vi "ReadTestConfig.vi"(11 "Model":string) -> (3 "TestItemsOut":string[][](table))   [LabVIEW 2009]
uses:
  <vilib>/Utility/file.llb/Read From Spreadsheet File (string).vi
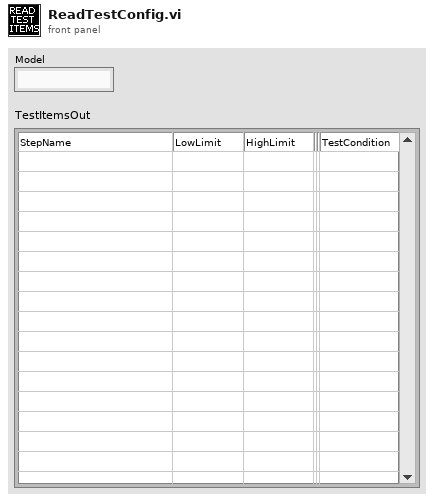
[diagram p1: front panel]
types:
  T1 = enum32{"invalid app kind", "Development System", "Run Time System", "Student Edition", "Embedded LabVIEW", "Evaluation", "Custom"}
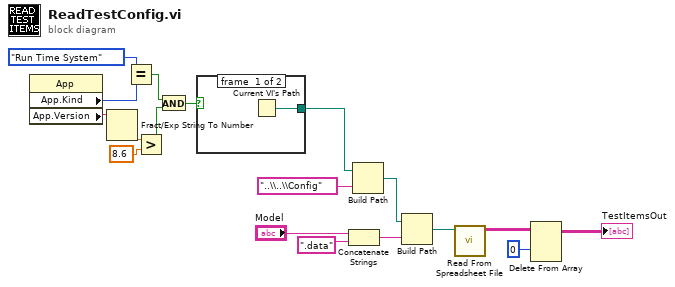
[diagram p0: block diagram]
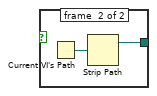
[diagram p2: hidden frame]
diagram:
  n1 = property class="App"() -> ("App.Kind"=w4:T1, "App.Version"=w5:string)  [unwired: 2 in, 2 out]
  n2 = Fract/Exp String To Number(string=w5) -> (number=w6:dbl)  [unwired: 4 out]
  n3 = Equal?(x=T1."Run Time System" ("y"), y=w4) -> (x = y?=w7:bool)
  n4 = Greater?(x=w6, y=8.6) -> (0:w8:bool)
  n5 = And(x=w7, y=w8) -> (x .and. y?=w2:bool)
  n6 = case shown="真" w2 {
    tunnel: [w19 w21] -> w17
    frame #0 {
      n7 = Current VI's Path() -> (path=w19:path)
    }
    frame #1 {
      n8 = Current VI's Path() -> (path=w20:path)
      n9 = Strip Path(path=w20) -> (stripped path=w21:path)  [unwired: 1 out]
    }
  }
  n10 = Concatenate Strings("Model", ".data" ("pattern (all files)")) -> (w12:string)
  n11 = Build Path(base path=w17, name or relative path="..\\..\\Config" ("名称或相对路径")) -> (appended path=w15:path)
  n12 = Build Path(base path=w15, name or relative path=w12) -> (appended path=w18:path)
  n13 = call-poly <vilib>:"Read From Spreadsheet File.vi"("file path (dialog if empty)"=w18) -> ("all rows"=w10:string[][])  [unwired: 3 in, 7 out]
  n14 = Delete From Array(array=w10, index (row)=0 ("索引 (行)")) -> (array with subset deleted=→"TestItemsOut":string[][])  [unwired: 2 in, 1 out]
